vi "theta_LP.vi"(2 "error in (no error)":errorcluster, 3 "th_in":T1, 4 "low cutoff freq: fl":dbl=0.125 format="%0.3f") -> (0 "error out":errorcluster, 1 "th_out":T1)   [LabVIEW 2021]
uses:
  <vilib>/Analysis/Matrix/Datatypes/RealMatrix.ctl
  <vilib>/Analysis/3filter.llb/Filter Passband Type.ctl
  <vilib>/ptbypt/NI_PtbyPt.lvlib
  <vilib>/Analysis/NI_AALBase.lvlib
  <vilib>/Analysis/Matrix/NI_Matrix.lvlib
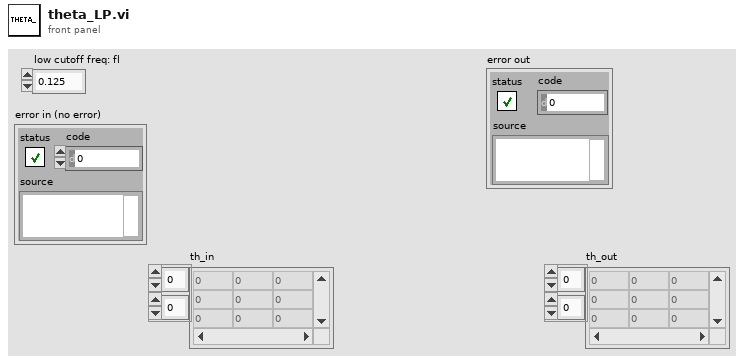
[diagram p1: front panel]
types:
  T1 = typedef "NI_Matrix.lvlib/RealMatrix.ctl" = dbl[][]
  T2 = typedef "NI_AALBase.lvlib/Filter Passband Type.ctl" = enum32{"Lowpass", "Highpass", "Bandpass", "Bandstop"}
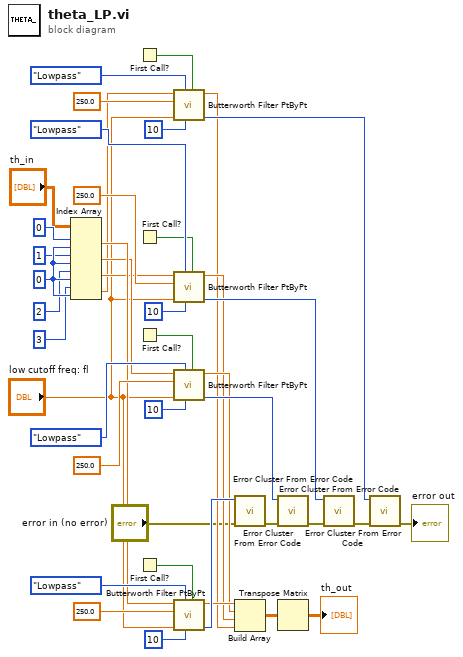
[diagram p0: block diagram]
diagram:
  w35 = 0 ("index (col)")
  n1 = Index Array(array="th_in", index (row) #1=0 ("index (row)"), index (col) #1=w35, index (row) #2=1 ("index (row)"), index (col) #2=w35, index (row) #3=2 ("index (row)"), index (col) #3=w35, index (row) #4=3 ("index (row)"), index (col) #4=w35) -> (element #1=w12:dbl, element #2=w10:dbl, element #3=w8:dbl, element #4=w6:dbl)
  n2 = First Call?() -> (First Call?: T/F=w18:bool)
  n3 = First Call?() -> (First Call?: T/F=w23:bool)
  n4 = First Call?() -> (First Call?: T/F=w28:bool)
  n5 = First Call?() -> (First Call?: T/F=w38:bool)
  n6 = call <vilib>:"Butterworth Filter PtByPt.vi"("initialize"=w18, "order"=10, "filter type"=Filter_Passband_Type."Lowpass", "low cutoff freq: fl"="low cutoff freq: fl", "sampling freq: fs"=250.0, "x"=w6) -> ("error"=w16:i32, "Filtered x"=w5:dbl)  [unwired: 3 in]
  n7 = call <vilib>:"Butterworth Filter PtByPt.vi"("initialize"=w23, "order"=10, "filter type"=Filter_Passband_Type."Lowpass", "low cutoff freq: fl"="low cutoff freq: fl", "sampling freq: fs"=250.0, "x"=w8) -> ("error"=w21:i32, "Filtered x"=w7:dbl)  [unwired: 3 in]
  n8 = call <vilib>:"Butterworth Filter PtByPt.vi"("initialize"=w28, "order"=10, "filter type"=Filter_Passband_Type."Lowpass", "low cutoff freq: fl"="low cutoff freq: fl", "sampling freq: fs"=250.0, "x"=w10) -> ("error"=w26:i32, "Filtered x"=w9:dbl)  [unwired: 3 in]
  n9 = call <vilib>:"Butterworth Filter PtByPt.vi"("initialize"=w38, "order"=10, "filter type"=Filter_Passband_Type."Lowpass", "low cutoff freq: fl"="low cutoff freq: fl", "sampling freq: fs"=250.0, "x"=w12) -> ("error"=w36:i32, "Filtered x"=w11:dbl)  [unwired: 3 in]
  n10 = call <vilib>:"Error Cluster From Error Code.vi"("error in (no error)"="error in (no error)", "error code (0)"=w36) -> ("error out"=w15:errorcluster)  [unwired: 7 in]
  n11 = Build Array(w11, w9, w7, w5) -> (w42:T1)
  n12 = call <vilib>:"Error Cluster From Error Code.vi"("error in (no error)"=w15, "error code (0)"=w26) -> ("error out"=w14:errorcluster)  [unwired: 7 in]
  n13 = Transpose Matrix(1:w42) -> (0:→"th_out":T1)
  n14 = call <vilib>:"Error Cluster From Error Code.vi"("error in (no error)"=w14, "error code (0)"=w21) -> ("error out"=w13:errorcluster)  [unwired: 7 in]
  n15 = call <vilib>:"Error Cluster From Error Code.vi"("error in (no error)"=w13, "error code (0)"=w16) -> ("error out"=→"error out":errorcluster)  [unwired: 7 in]
